vi "test.vi"() -> ()   [LabVIEW 2016]
uses:
  <vilib>/ptbypt/NI_PtbyPt.lvlib
panel:
  out "周期设置 2":cluster{"启动":bool, "控制命令":T1}
  out "数值":i32
  out "间隔计时":dbl
  out "启动次数":i32
  out "仪器运行状态":bool
  out "最近一次结束时间":timestamp
  out "最近一次启动时间":timestamp
  in  "周期设置":cluster{"启动":bool, "控制命令":T1, "测量参数":T2}(xcontrol)
  in  "仪器运行状态 2":bool
  out "数组":T3(array[cluster])
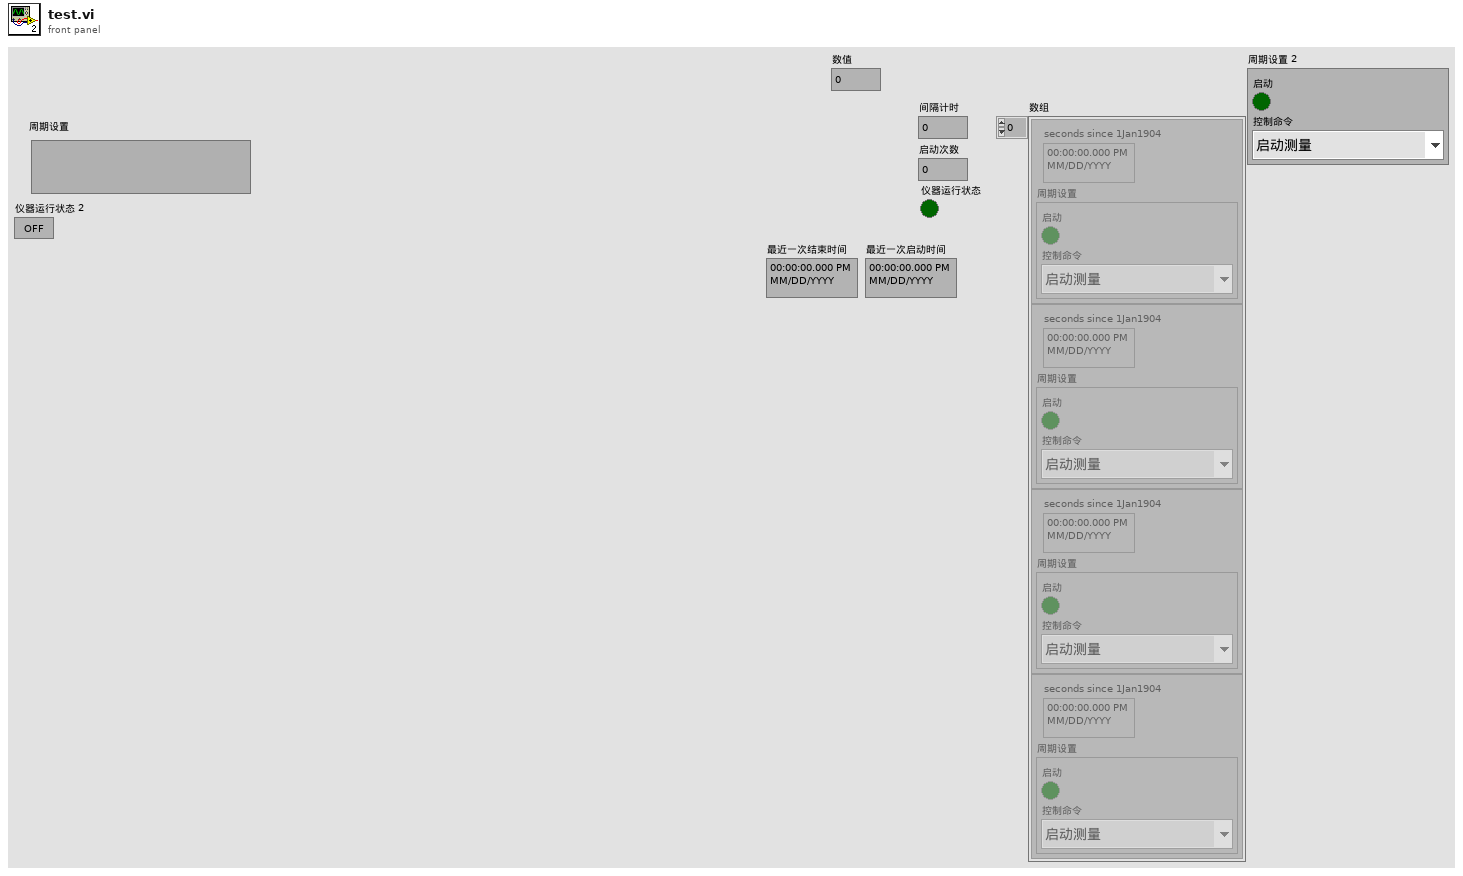
[diagram p1: front panel]
types:
  T1 = typedef "定时设置.xctl/国标控制命令.ctl" = enum16{"启动测量", "标样核查", "零点核查", "跨度核查", "空白测试", "平行样测试", "加标回收", "空白校准", "标样校准", "初始化（清洗）", "停止测试", "仪器重启", "校时", "模式设置", "测量间隔设置"}
  T2 = typedef "定时设置.xctl/测量参数.ctl" = u16
  T3 = cluster{"seconds since 1Jan1904":timestamp, "周期设置":cluster{"启动":bool, "控制命令":T1}}[]
  T4 = typedef "定时设置.xctl/周期模式设置.ctl" = enum16{"不启用", "定点模式", "间隔模式"}
  T5 = typedef "定时设置.xctl/定点周期设置.ctl" = cluster{"启动命令":T6, "启动命令 2":T6, "启动命令 3":T6, "启动命令 4":T6, "启动命令 5":T6, "启动命令 6":T6, "启动命令 7":T6, "启动命令 8":T6, "启动命令 9":T6, "启动命令 10":T6, "启动命令 11":T6, "启动命令 12":T6, "启动命令 13":T6, "启动命令 14":T6, "启动命令 15":T6, "启动命令 16":T6, "启动命令 17":T6, "启动命令 18":T6, "启动命令 19":T6, "启动命令 20":T6, "启动命令 21":T6, "启动命令 22":T6, "启动命令 23":T6, "启动命令 24":T6}
  T6 = typedef "定时设置.xctl/启动命令选择.ctl" = u16
  T7 = typedef "定时设置.xctl/间隔启动设置.ctl" = cluster{"启动命令":T6, "启动间隔":dbl, "启动次数":i32}
  T8 = cluster{"周期模式":T4, "定点周期":T5, "间隔启动":T7, "测量参数":T2}
  T9 = cluster{"seconds since 1Jan1904":timestamp, "周期设置":cluster{"启动":bool, "控制命令":T1, "测量参数":T2}}
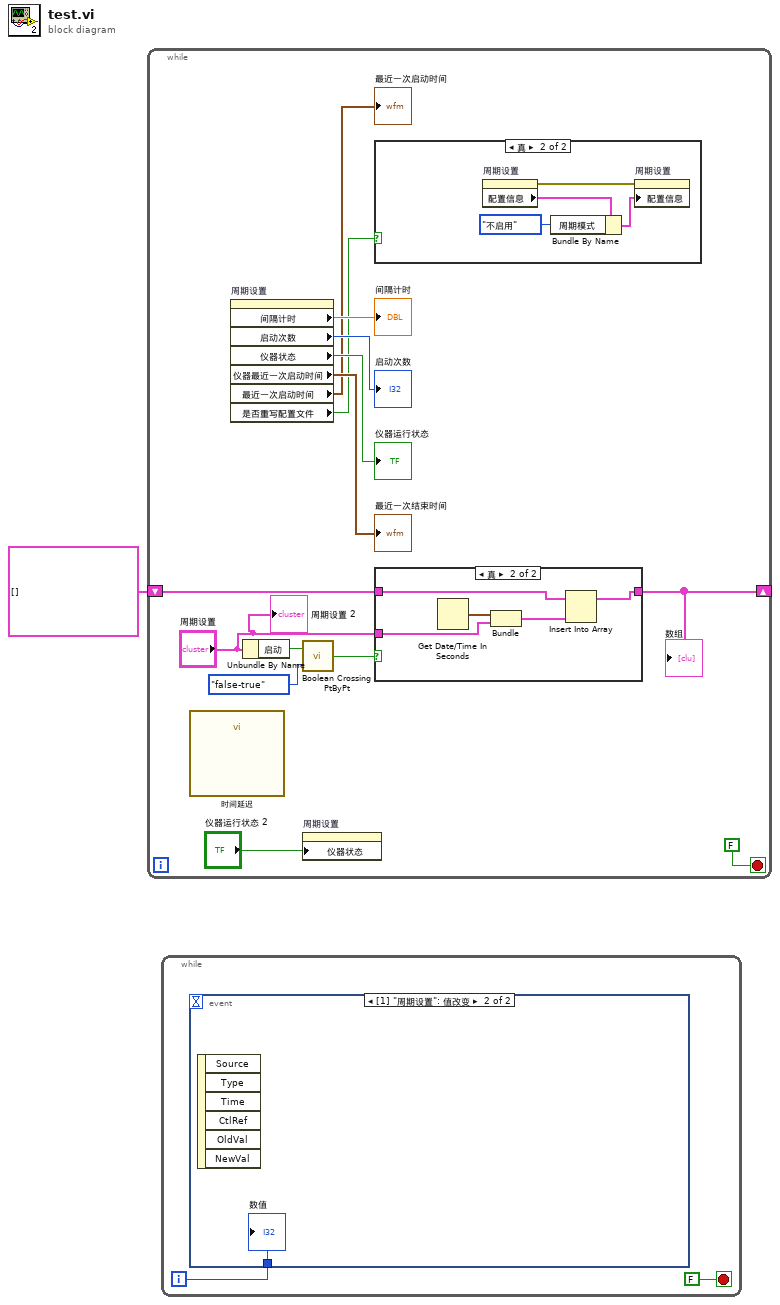
[diagram p0: block diagram]
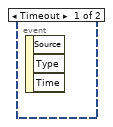
[diagram p2: hidden frame]
diagram:
  n1 = while {
    shift-right: [w6] -> _
    shift-left: T3 [] -> [w5]
    stop <- FALSE stop-if-true
    n2 = call "时间延迟"() -> ()  [unwired: 11 in, 1 out]
    n3 = property on="周期设置" class="定时设置 (严格)"() -> ("间隔计时"=→"间隔计时":dbl, "启动次数"=→"启动次数":i32, "仪器状态"=→"仪器运行状态":bool, "仪器最近一次启动时间"=→"最近一次结束时间":timestamp, "最近一次启动时间"=→"最近一次启动时间":timestamp, "是否重写配置文件"=w3:bool)  [unwired: 2 in, 2 out]
    n4 = Unbundle By Name("周期设置") -> ("启动"=w9:bool)
    n5 = call <vilib>:"Boolean Crossing PtByPt.vi"("direction"=enum16{"either", "false-true", "true-false"}."false-true", "input"=w9) -> ("crossing"=w7:bool)  [unwired: 1 in]
    n6 = property on="周期设置" class="定时设置 (严格)"("仪器状态"="仪器运行状态 2") -> ()  [unwired: 2 in, 2 out]
    n7 = case shown="真" w3 {
      frame False {
      }
      frame True {
        n8 = property on="周期设置" class="定时设置 (严格)"() -> (error out=w19:errorcluster, "配置信息"=w18:T8)  [unwired: 2 in, 1 out]
        n9 = Bundle By Name(cluster=w18, "周期模式"=周期模式设置."不启用") -> (w17:T8)
        n10 = property on="周期设置" class="定时设置 (严格)"(error in=w19, "配置信息"=w17) -> ()  [unwired: 1 in, 2 out]
      }
    }
    n11 = case shown="真" w7 {
      tunnel: "周期设置" -> [_ w24]
      tunnel: [w20 w22] -> w6
      tunnel: w5 -> [w20 w21]
      frame False {
      }
      frame True {
        n12 = Get Date/Time In Seconds() -> (seconds since 1Jan1904=w25:timestamp)
        n13 = Bundle("seconds since 1Jan1904"=w25, "周期设置"=w24) -> (w23:T9)  [unwired: 1 in]
        n14 = Insert Into Array(array=w21, new element=w23) -> (w22:T3)  [unwired: 1 in]
      }
    }
    "数组" <- w6
    "周期设置 2" <- "周期设置"
  }
  n15 = while {
    i -> [w26]
    stop <- FALSE stop-if-true
    n16 = event shown="[1] \"周期设置\": 值改变" {
      selector: _ -> [_ _]
      dyn-events: _ -> [_ _]
      timeout: _ -> [_ _]
      tunnel: w26 -> [_ w28]
      event Timeout {
        n17 = event-data() -> ()  [unwired: 1 in, 3 out]
      }
      event "周期设置": Value Change {
        n18 = event-data() -> ()  [unwired: 1 in, 6 out]
        "数值" <- w28
      }
    }
  }
